vi "MSScript_Transform_EXTArray.vi"(5 "upper limit (Inf)":ext=inf, 7 "lower limit (-Inf)":ext=-inf, 8 "MinSize":i32=-1, 9 "MaxSize":i32=-1, 11 "check_str":string="0 1 2") -> (1 "Is a variable ?":bool, 2 "Value Error?":bool, 3 "Value Output":ext[](array[numeric])=[0.0, 1.0, 2.0])   [LabVIEW 2018, in "MSScript.lvclass"]
uses:
  MSScript.lvclass
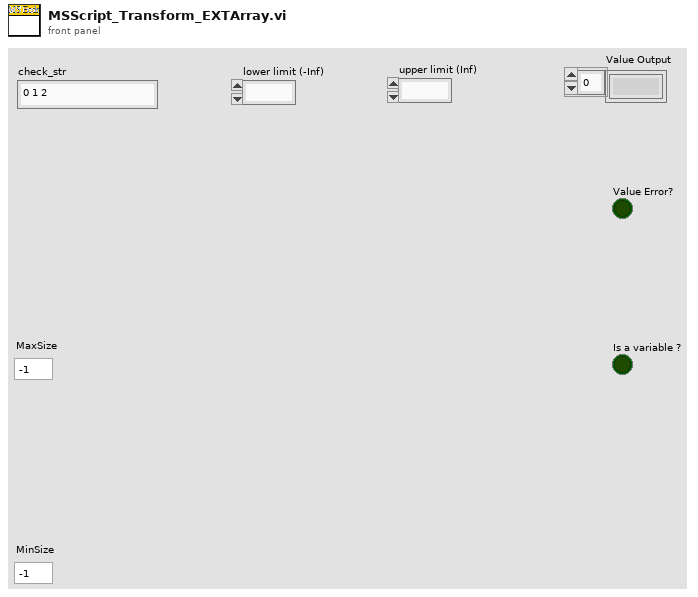
[diagram p1: front panel]
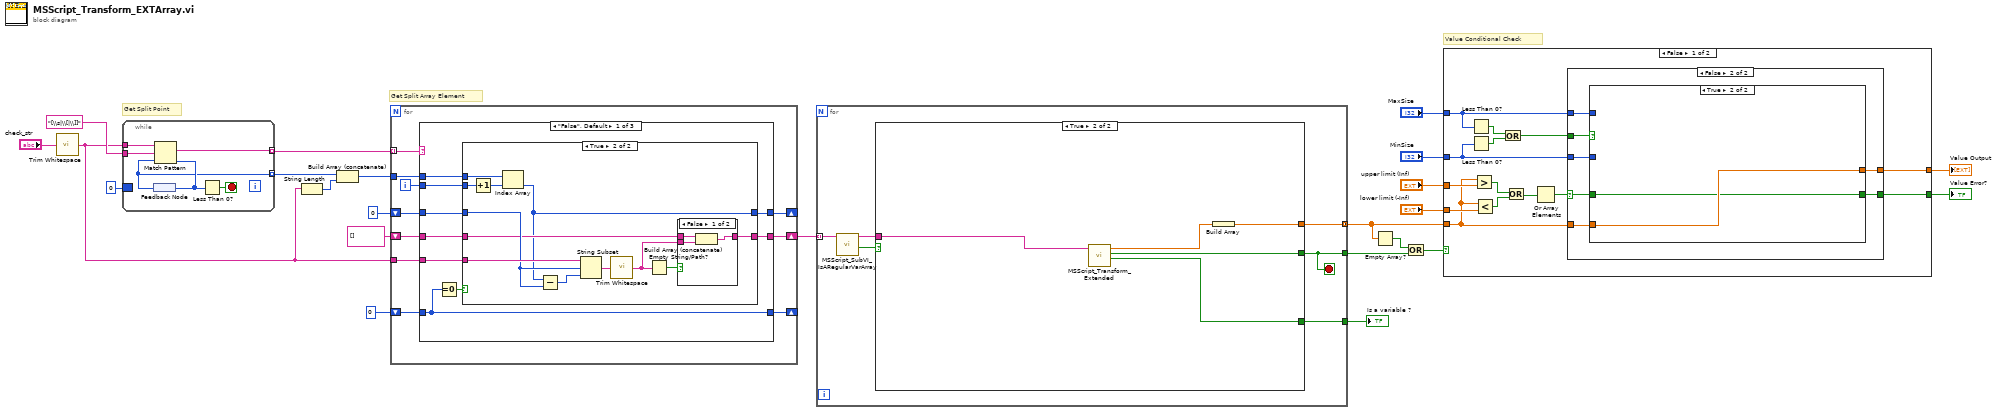
[diagram p0: block diagram]
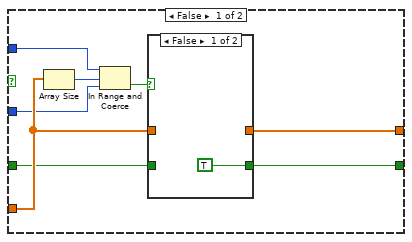
[diagram p3: hidden frame]
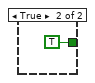
[diagram p5: hidden frame]
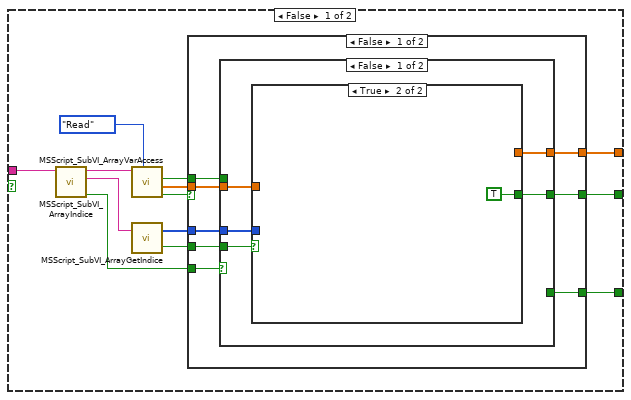
[diagram p6: hidden frame]
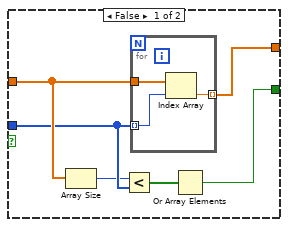
[diagram p7: hidden frame]
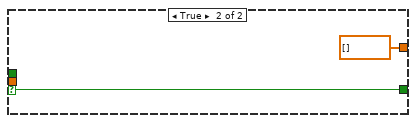
[diagram p9: hidden frame]
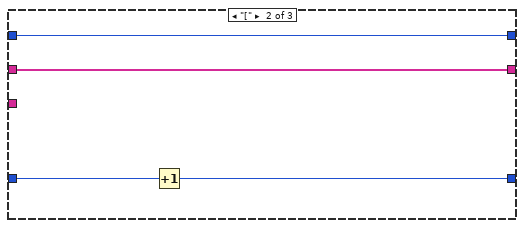
[diagram p12: hidden frame]
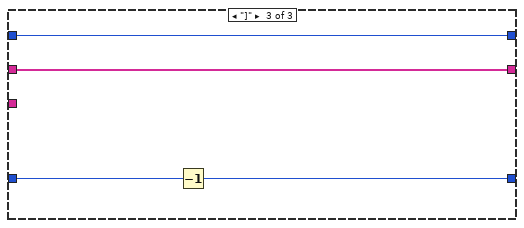
[diagram p13: hidden frame]
diagram:
  # "Value Conditional Check"
  # "Get Split Array Element"
  # "Get Split Point"
  n1 = call <vilib>:"Trim Whitespace.vi"("string"="check_str") -> ("trimmed string"=w13:string)  [unwired: 1 in]
  n2 = while {
    tunnel: w13 -> [w29]
    tunnel: [w28] -> w7 mode=indexing
    border: 0 ("offset past match") -> [_]
    tunnel: "[\\s|\\[|\\]]" ("regular expression") -> [w25]
    tunnel: [w24] -> w12 mode=indexing
    stop <- w27 stop-if-true
    n3 = feedback #1() -> (w24:i32)
    n4 = Match Pattern(string=w29, regular expression=w25, offset (0)=w24) -> (match substring=w28:string, offset past match=w26:i32)  [unwired: 2 out]
    n5 = feedback-in #1(w26) -> ()
    n6 = Less Than 0?(x=w26) -> (x < 0?=w27:bool)
  }
  n7 = String Length(string=w13) -> (length=w11:i32)
  n8 = Build Array (concatenate)(w12, w11) -> (w10:i32[])
  n9 = for {
    tunnel: w7 -> [w39] mode=indexing
    tunnel: w10 -> [w36]
    shift-right: [w37] -> _
    shift-left: 0 -> [w38]
    tunnel: w13 -> [w34]
    shift-right: [w32] -> _
    shift-left: 0 -> [w33]
    shift-right: [w31] -> w6
    shift-left: string[] [] -> [w30]
    i -> [w35]
    n10 = case shown="\"False\", Default" w39 {
      tunnel: w38 -> [w48 w70 w74]
      tunnel: [w48 w69 w73] -> w37
      tunnel: w36 -> [w46 _ _]
      tunnel: w35 -> [w45 _ _]
      tunnel: w34 -> [w44 _ _]
      tunnel: w33 -> [w43 w68 w72]
      tunnel: [w42 w68 w72] -> w32
      tunnel: [w41 w67 w71] -> w31
      tunnel: w30 -> [w40 w67 w71]
      frame "False", Default {
        n11 = Equal To 0?(x=w48) -> (x = 0?=w47:bool)
        n12 = case shown="True" w47 {
          tunnel: w46 -> [_ w62]
          tunnel: w45 -> [_ w60]
          tunnel: w44 -> [_ w61]
          tunnel: w43 -> [w49 w58]
          tunnel: [w49 w54] -> w42
          tunnel: [w50 w56] -> w41
          tunnel: w40 -> [w50 w55]
          frame False {
          }
          frame True {
            n13 = Increment(x=w60) -> (x+1=w59:i32)
            n14 = Index Array(array=w62, index=w59) -> (element=w54:i32)
            n15 = Subtract(x=w54, y=w58) -> (x-y=w57:i32)
            n16 = String Subset(string=w61, offset (0)=w58, length (rest)=w57) -> (substring=w52:string)
            n17 = call <vilib>:"Trim Whitespace.vi"("string"=w52) -> ("trimmed string"=w51:string)  [unwired: 1 in]
            n18 = Empty String/Path?(string/path=w51) -> (empty?=w53:bool)
            n19 = case shown="False" w53 {
              tunnel: [w65 w66] -> w56
              tunnel: w55 -> [w64 w66]
              tunnel: w51 -> [w63 _]
              frame False {
                n20 = Build Array (concatenate)(w64, w63) -> (w65:string[])
              }
              frame True {
              }
            }
          }
        }
      }
      frame "[" {
        n21 = Increment(x=w70) -> (x+1=w69:i32)
      }
      frame "]" {
        n22 = Decrement(x=w74) -> (x-1=w73:i32)
      }
    }
  }
  n23 = for {
    tunnel: w6 -> [w80] mode=indexing
    tunnel: [w77] -> w3 mode=concatenating
    tunnel: [w76] -> w4
    tunnel: [w75] -> w1
    stop <- w76 stop-if-true
    n24 = call "MSScript_SubVI_IsARegularVarArray.vi"("VarString in"=w80) -> ("Variable simbol no found"=w78:bool, "VarString out"=w79:string)  [unwired: 6 in, 1 out]
    n25 = case shown="True" w78 {
      tunnel: [w91 w124] -> w77
      tunnel: [w89 w123] -> w76
      tunnel: w79 -> [w83 w122]
      tunnel: [w81 w121] -> w75
      frame False {
        n26 = call "MSScript_SubVI_ArrayIndice.vi"("@name[x:y|z]"=w83) -> ("Index no found"=w87:bool, "Indice string"=w86:string, "@name"=w92:string)  [unwired: 6 in]
        n27 = call "MSScript_SubVI_ArrayVarAccess.vi"("Function (Read)"=enum16{"Init", "Write", "Read"}."Read", "VarName"=w92) -> ("Value Error?"=w88:bool, "ArrayVariable out"=w90:ext[], "Is a variable ?"=w82:bool)  [unwired: 5 in]
        n28 = call "MSScript_SubVI_ArrayGetIndice.vi"("indice string in"=w86) -> ("error"=w84:bool, "x:y"=w85:i32[])  [unwired: 1 in]
        n29 = case shown="False" w88 {
          selector: w88 -> [_ w119]
          tunnel: w87 -> [w101 _]
          tunnel: [w100 ext[] [] ("ArrayVariable out")] -> w91
          tunnel: w90 -> [w99 _]
          tunnel: [w98 w119] -> w89
          tunnel: w85 -> [w97 _]
          tunnel: w84 -> [w96 _]
          tunnel: w82 -> [w95 _]
          tunnel: [w94 _] -> w81
          frame False {
            n30 = case shown="False" w101 {
              tunnel: [w105 w118] -> w100
              tunnel: w99 -> [w106 w118]
              tunnel: [w104 _] -> w98
              tunnel: w97 -> [w103 _]
              tunnel: w96 -> [w102 _]
              tunnel: w95 -> [_ w117]
              tunnel: [_ w117] -> w94
              frame False {
                n31 = case shown="True" w102 {
                  tunnel: w106 -> [w111 _]
                  tunnel: [w112 _] -> w105
                  tunnel: [w108 TRUE ("Value Error?")] -> w104
                  tunnel: w103 -> [w110 _]
                  frame False {
                    n32 = Array Size(array=w111) -> (size(s)=w107:i32)
                    n33 = Less?(x=w107, y=w110) -> (x < y?=w109:bool[])
                    n34 = for {
                      tunnel: w110 -> [w115] mode=indexing
                      tunnel: w111 -> [w114]
                      tunnel: [w113] -> w112 mode=indexing
                      n35 = Index Array(array=w114, index=w115) -> (element=w113:ext)
                    }
                    n36 = Or Array Elements(Boolean array=w109) -> (logical OR=w108:bool)
                  }
                  frame True {
                  }
                }
              }
              frame True {
              }
            }
          }
          frame True {
          }
        }
      }
      frame True {
        n37 = call "MSScript_Transform_Extended.vi"("Check_Str"=w122) -> ("Is a variable ?"=w121:bool, "Value Error?"=w123:bool, "Value Output"=w125:ext)  [unwired: 8 in]
        n38 = Build Array(w125) -> (w124:ext[])
      }
    }
  }
  "Is a variable ?" <- w1
  n39 = Empty Array?(array=w3) -> (empty?=w5:bool)
  n40 = Or(x=w5, y=w4) -> (x .or. y?=w2:bool)
  n41 = case shown="False" w2 {
    tunnel: [w139 TRUE] -> w23
    tunnel: "MaxSize" -> [w138 _]
    tunnel: "MinSize" -> [w137 _]
    tunnel: [w133 _] -> w20
    tunnel: "upper limit (Inf)" -> [w129 _]
    tunnel: "lower limit (-Inf)" -> [w128 _]
    tunnel: w3 -> [w127 _]
    frame False {
      n42 = Less Than 0?(x=w138) -> (x < 0?=w135:bool)
      n43 = Less Than 0?(x=w137) -> (x < 0?=w136:bool)
      n44 = Greater?(x=w127, y=w129) -> (0:w132:bool[])
      n45 = Less?(x=w127, y=w128) -> (x < y?=w131:bool[])
      n46 = Or(x=w135, y=w136) -> (x .or. y?=w134:bool)
      n47 = Or(x=w132, y=w131) -> (x .or. y?=w130:bool[])
      n48 = Or Array Elements(Boolean array=w130) -> (logical OR=w126:bool)
      n49 = case shown="False" w126 {
        selector: w126 -> [w140 w141]
        tunnel: w127 -> [_ w147]
        tunnel: [w140 w146] -> w139
        tunnel: w138 -> [_ w145]
        tunnel: w137 -> [_ w144]
        tunnel: w134 -> [_ w143]
        tunnel: [_ w142] -> w133
        frame True {
        }
        frame False {
          n50 = case shown="True" w143 {
            tunnel: w147 -> [w154 w160]
            tunnel: [w152 w159] -> w146
            tunnel: w145 -> [w151 _]
            tunnel: w144 -> [w150 _]
            tunnel: [w149 w160] -> w142
            tunnel: w141 -> [w148 w159]
            frame False {
              n51 = Array Size(array=w154) -> (size(s)=w155:i32)
              n52 = In Range and Coerce(upper limit=w151, x=w155, lower limit=w150) -> (In Range?=w153:bool)  [unwired: 1 out]
              n53 = case shown="False" w153 {
                tunnel: w154 -> [_ w158]
                tunnel: [TRUE w157] -> w152
                tunnel: [_ w158] -> w149
                tunnel: w148 -> [_ w157]
                frame False {
                }
                frame True {
                }
              }
            }
            frame True {
            }
          }
        }
      }
    }
    frame True {
    }
  }
  "Value Error?" <- w23
  "Value Output" <- w20
